vi "webrelay.vi"() -> ()   [LabVIEW 2021]
panel:
  in  "?":enum32{"Network Settings", "Control"}(tab)
  in  "Port":u16=80
  in  "Address":string
  in  "?":bool
  in  "?":bool
  in  "?":bool
  out "Input State":string
  out "Relay State":string
  # "Webrelay Control Demo - LabVIEW"
  # "Set the IP Address and Port number of the Webrelay unit that will be monitored and controlled."
  # "Monitor the state of the Webrelay unit on the left. Control the state of the relay with the buttons above."
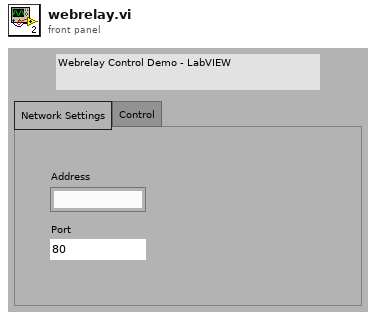
[diagram p1: front panel]
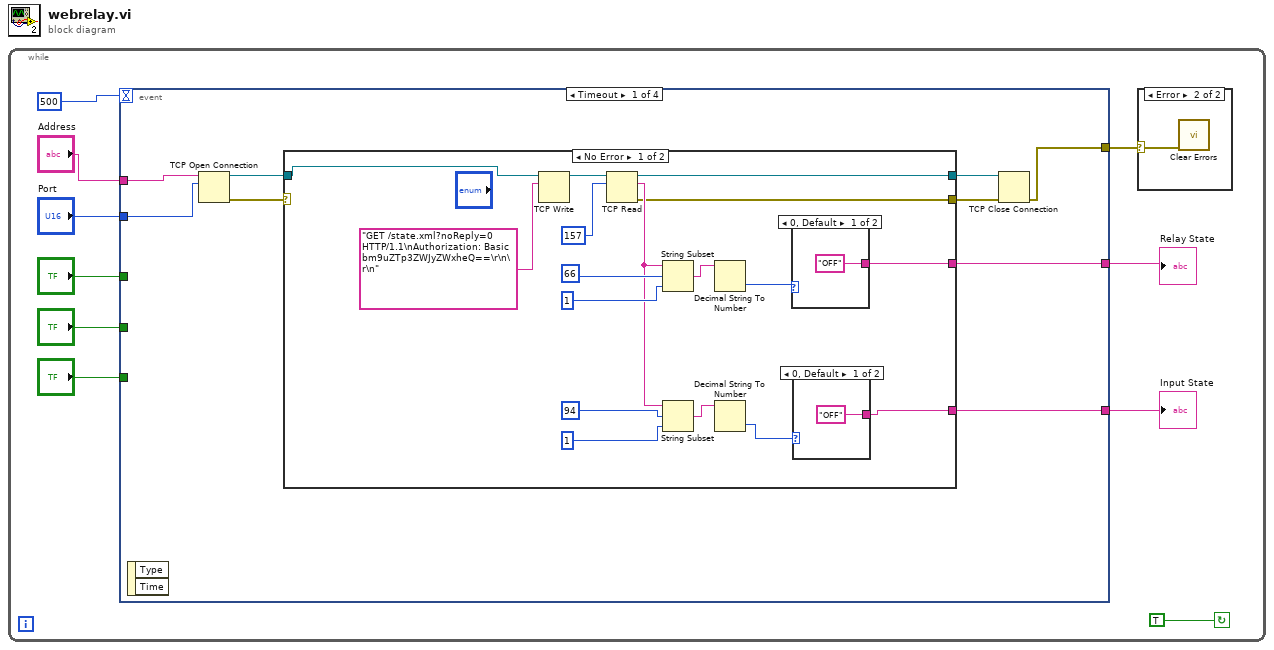
[diagram p0: block diagram]
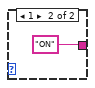
[diagram p3: hidden frame]
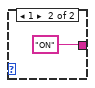
[diagram p4: hidden frame]
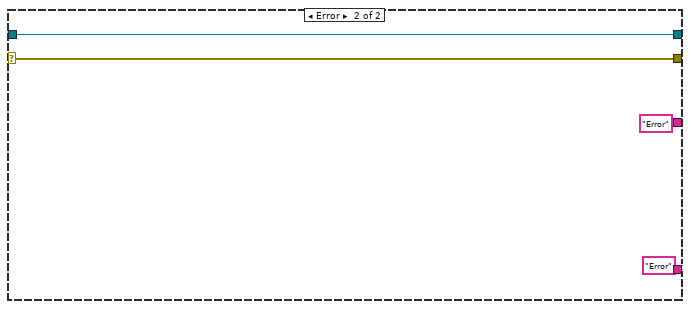
[diagram p5: hidden frame]
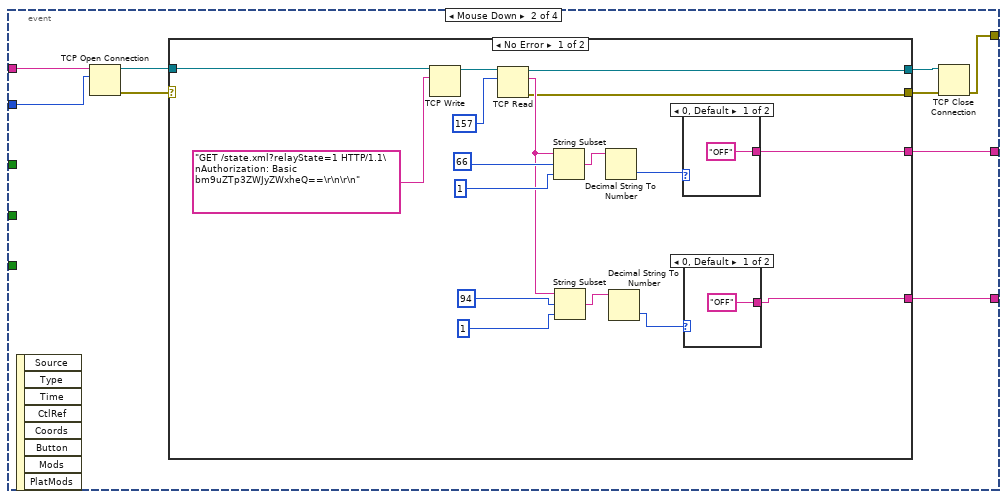
[diagram p6: hidden frame]
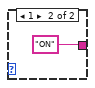
[diagram p7: hidden frame]
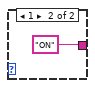
[diagram p8: hidden frame]
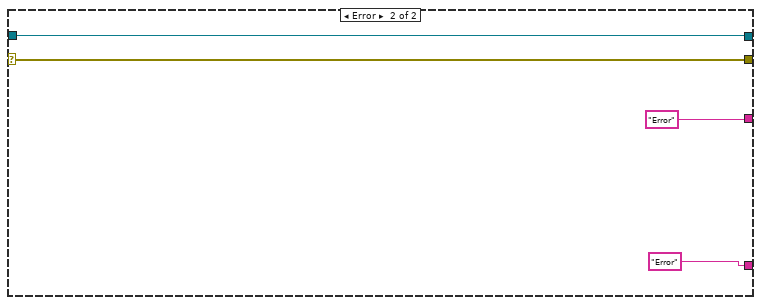
[diagram p9: hidden frame]
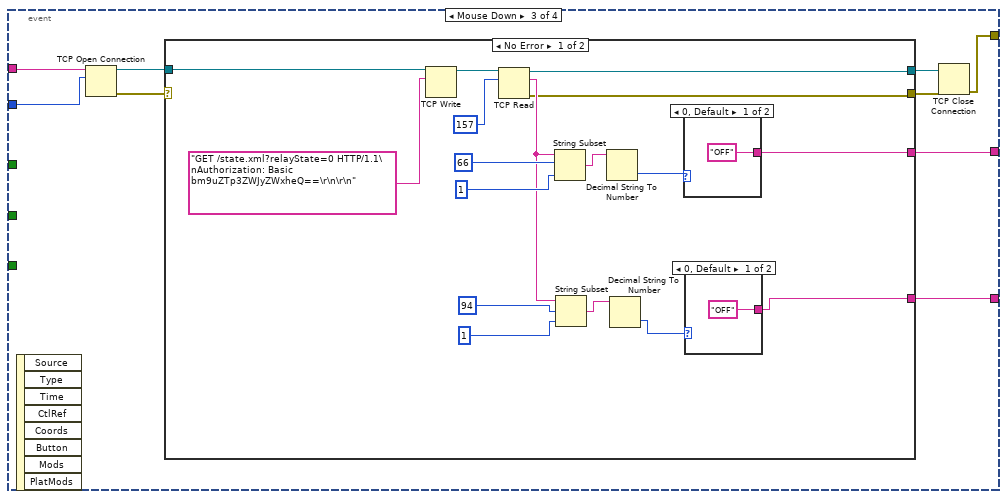
[diagram p10: hidden frame]
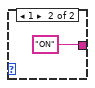
[diagram p11: hidden frame]
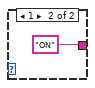
[diagram p12: hidden frame]
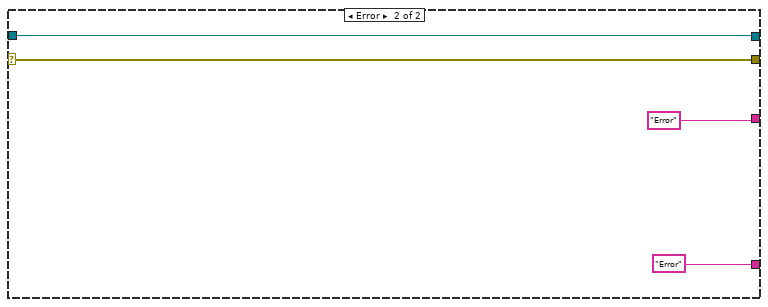
[diagram p13: hidden frame]
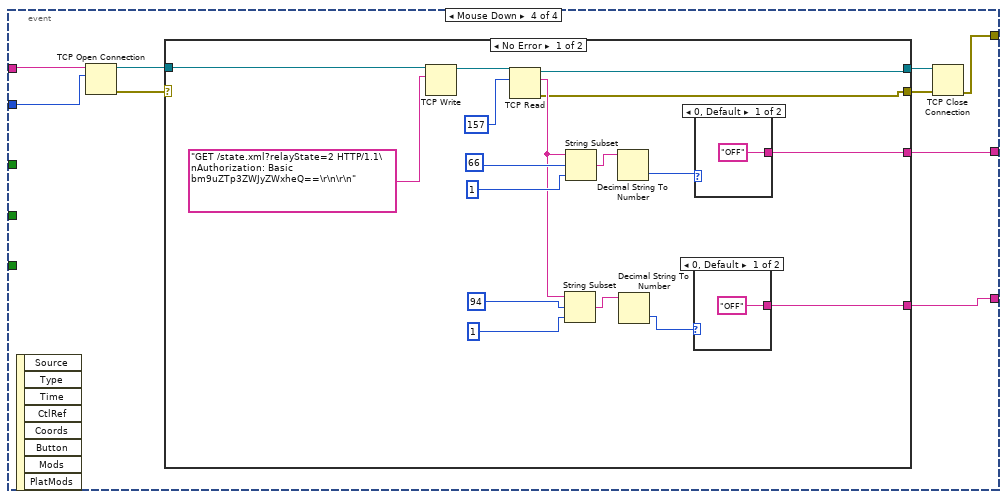
[diagram p14: hidden frame]
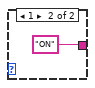
[diagram p15: hidden frame]
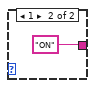
[diagram p16: hidden frame]
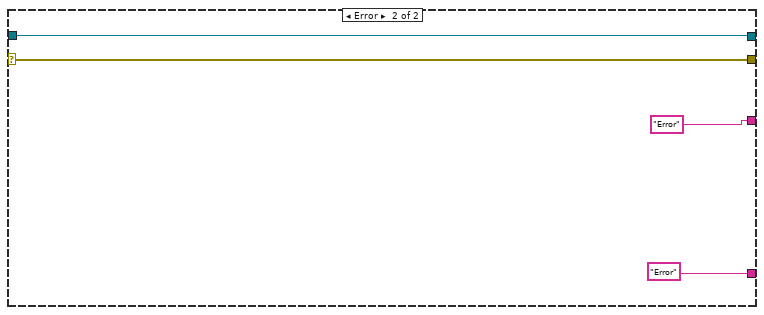
[diagram p17: hidden frame]
diagram:
  n1 = while {
    stop <- TRUE continue-if-true
    n2 = event shown="[0] Timeout" {
      selector: _ -> [_ _ _ _]
      dyn-events: _ -> [_ _ _ _]
      timeout: 500 -> [_ _ _ _]
      tunnel: "Address" -> [w20 w52 w86 w120]
      tunnel: "Port" -> [w19 w51 w85 w119]
      tunnel: "?" -> [_ _ _ _]
      tunnel: "?" -> [_ _ _ _]
      tunnel: "?" -> [_ _ _ _]
      tunnel: [w18 w50 w84 w118] -> w4
      tunnel: [w17 w49 w83 w117] -> w3
      tunnel: [w12 w46 w80 w114] -> w1
      event Timeout {
        n3 = event-data() -> ()  [unwired: 1 in, 2 out]
        n4 = TCP Open Connection(address=w20, remote port or service name=w19) -> (connection ID=w13:refnum<k5>, error out=w14:errorcluster)  [unwired: 3 in]
        n5 = case shown="No Error" w14 {
          selector: w14 -> [_ w43]
          tunnel: [w30 "Error"] -> w18
          tunnel: [w26 "Error"] -> w17
          tunnel: [w23 w43] -> w16
          tunnel: [w22 w42] -> w15
          tunnel: w13 -> [w21 w42]
          frame No Error {
            n6 = TCP Write(connection ID=w21, data in="GET /state.xml?noReply=0 HTTP/1.1\nAuthorization: Basic bm9uZTp3ZWJyZWxheQ==\r\n\r\n") -> (connection ID out=w36:refnum<k5>)  [unwired: 2 in, 2 out]
            n7 = TCP Read(connection ID=w36, bytes to read=157) -> (connection ID out=w22:refnum<k5>, data out=w29:string, error out=w23:errorcluster)  [unwired: 3 in]
            n8 = String Subset(string=w29, offset (0)=66, length (rest)=1) -> (substring=w32:string)
            n9 = String Subset(string=w29, offset (0)=94, length (rest)=1) -> (substring=w25:string)
            n10 = Decimal String To Number(string=w32) -> (number=w31:i32)  [unwired: 2 in, 1 out]
            n11 = Decimal String To Number(string=w25) -> (number=w24:i32)  [unwired: 2 in, 1 out]
            n12 = case shown="0, Default" w31 {
              tunnel: ["OFF" "ON"] -> w30
              frame 0, Default {
              }
              frame 1 {
              }
            }
            n13 = case shown="0, Default" w24 {
              tunnel: ["OFF" "ON"] -> w26
              frame 0, Default {
              }
              frame 1 {
              }
            }
          }
          frame Error {
          }
        }
        n14 = TCP Close Connection(connection ID=w15, error in (no error)=w16) -> (error out=w12:errorcluster)  [unwired: 1 in, 1 out]
      }
      event Mouse Down {
        n15 = event-data() -> ()  [unwired: 1 in, 8 out]
        n16 = TCP Open Connection(address=w52, remote port or service name=w51) -> (connection ID=w53:refnum<k5>, error out=w54:errorcluster)  [unwired: 3 in]
        n17 = case shown="No Error" w54 {
          selector: w54 -> [_ w76]
          tunnel: w53 -> [w71 w79]
          tunnel: [w67 w79] -> w48
          tunnel: [w62 "Error"] -> w50
          tunnel: [w58 "Error"] -> w49
          tunnel: [w55 w76] -> w47
          frame No Error {
            n18 = TCP Write(connection ID=w71, data in="GET /state.xml?relayState=1 HTTP/1.1\nAuthorization: Basic bm9uZTp3ZWJyZWxheQ==\r\n\r\n") -> (connection ID out=w69:refnum<k5>)  [unwired: 2 in, 2 out]
            n19 = TCP Read(connection ID=w69, bytes to read=157) -> (connection ID out=w67:refnum<k5>, data out=w61:string, error out=w55:errorcluster)  [unwired: 3 in]
            n20 = String Subset(string=w61, offset (0)=66, length (rest)=1) -> (substring=w64:string)
            n21 = String Subset(string=w61, offset (0)=94, length (rest)=1) -> (substring=w57:string)
            n22 = Decimal String To Number(string=w64) -> (number=w63:i32)  [unwired: 2 in, 1 out]
            n23 = Decimal String To Number(string=w57) -> (number=w56:i32)  [unwired: 2 in, 1 out]
            n24 = case shown="0, Default" w63 {
              tunnel: ["OFF" "ON"] -> w62
              frame 0, Default {
              }
              frame 1 {
              }
            }
            n25 = case shown="0, Default" w56 {
              tunnel: ["OFF" "ON"] -> w58
              frame 0, Default {
              }
              frame 1 {
              }
            }
          }
          frame Error {
          }
        }
        n26 = TCP Close Connection(connection ID=w48, error in (no error)=w47) -> (error out=w46:errorcluster)  [unwired: 1 in, 1 out]
      }
      event Mouse Down {
        n27 = event-data() -> ()  [unwired: 1 in, 8 out]
        n28 = TCP Open Connection(address=w86, remote port or service name=w85) -> (connection ID=w87:refnum<k5>, error out=w88:errorcluster)  [unwired: 3 in]
        n29 = case shown="No Error" w88 {
          selector: w88 -> [_ w110]
          tunnel: w87 -> [w105 w113]
          tunnel: [w98 w113] -> w82
          tunnel: [w97 "Error"] -> w84
          tunnel: [w90 "Error"] -> w83
          tunnel: [w89 w110] -> w81
          frame No Error {
            n30 = TCP Write(connection ID=w105, data in="GET /state.xml?relayState=0 HTTP/1.1\nAuthorization: Basic bm9uZTp3ZWJyZWxheQ==\r\n\r\n") -> (connection ID out=w99:refnum<k5>)  [unwired: 2 in, 2 out]
            n31 = TCP Read(connection ID=w99, bytes to read=157) -> (connection ID out=w98:refnum<k5>, data out=w91:string, error out=w89:errorcluster)  [unwired: 3 in]
            n32 = String Subset(string=w91, offset (0)=66, length (rest)=1) -> (substring=w101:string)
            n33 = String Subset(string=w91, offset (0)=94, length (rest)=1) -> (substring=w93:string)
            n34 = Decimal String To Number(string=w101) -> (number=w100:i32)  [unwired: 2 in, 1 out]
            n35 = Decimal String To Number(string=w93) -> (number=w92:i32)  [unwired: 2 in, 1 out]
            n36 = case shown="0, Default" w100 {
              tunnel: ["OFF" "ON"] -> w97
              frame 0, Default {
              }
              frame 1 {
              }
            }
            n37 = case shown="0, Default" w92 {
              tunnel: ["OFF" "ON"] -> w90
              frame 0, Default {
              }
              frame 1 {
              }
            }
          }
          frame Error {
          }
        }
        n38 = TCP Close Connection(connection ID=w82, error in (no error)=w81) -> (error out=w80:errorcluster)  [unwired: 1 in, 1 out]
      }
      event Mouse Down {
        n39 = event-data() -> ()  [unwired: 1 in, 8 out]
        n40 = TCP Open Connection(address=w120, remote port or service name=w119) -> (connection ID=w121:refnum<k5>, error out=w122:errorcluster)  [unwired: 3 in]
        n41 = case shown="No Error" w122 {
          selector: w122 -> [_ w144]
          tunnel: w121 -> [w139 w147]
          tunnel: [w132 w147] -> w116
          tunnel: [w131 "Error"] -> w118
          tunnel: [w125 "Error"] -> w117
          tunnel: [w123 w144] -> w115
          frame No Error {
            n42 = TCP Write(connection ID=w139, data in="GET /state.xml?relayState=2 HTTP/1.1\nAuthorization: Basic bm9uZTp3ZWJyZWxheQ==\r\n\r\n") -> (connection ID out=w133:refnum<k5>)  [unwired: 2 in, 2 out]
            n43 = TCP Read(connection ID=w133, bytes to read=157) -> (connection ID out=w132:refnum<k5>, data out=w124:string, error out=w123:errorcluster)  [unwired: 3 in]
            n44 = String Subset(string=w124, offset (0)=94, length (rest)=1) -> (substring=w127:string)
            n45 = String Subset(string=w124, offset (0)=66, length (rest)=1) -> (substring=w135:string)
            n46 = Decimal String To Number(string=w135) -> (number=w134:i32)  [unwired: 2 in, 1 out]
            n47 = Decimal String To Number(string=w127) -> (number=w126:i32)  [unwired: 2 in, 1 out]
            n48 = case shown="0, Default" w126 {
              tunnel: ["OFF" "ON"] -> w125
              frame 0, Default {
              }
              frame 1 {
              }
            }
            n49 = case shown="0, Default" w134 {
              tunnel: ["OFF" "ON"] -> w131
              frame 0, Default {
              }
              frame 1 {
              }
            }
          }
          frame Error {
          }
        }
        n50 = TCP Close Connection(connection ID=w116, error in (no error)=w115) -> (error out=w114:errorcluster)  [unwired: 1 in, 1 out]
      }
    }
    "Relay State" <- w4
    "Input State" <- w3
    n51 = case shown="Error" w1 {
      selector: w1 -> [_ w11]
      frame No Error {
      }
      frame Error {
        n52 = call <vilib>:"Clear Errors.vi"("error in (no error)"=w11) -> ()  [unwired: 5 in, 2 out]
      }
    }
  }
